vi "12_final.vi"() -> ()   [LabVIEW 2023]
uses:
  <vilib>/Utility/file.llb/Write Delimited Spreadsheet (string).vi
  <vilib>/Utility/file.llb/Read Delimited Spreadsheet (string).vi
panel:
  out "array w/ subset deleted":string[][](array[string])
  out "all rows":string[][](array[string])
  in  "Listbox":i32(listbox)
  in  "stop":bool
  in  "citire":bool
  in  "l":dbl
  in  "L":dbl
  in  "salveaza":bool
  out "XY Graph":cluster{dbl[], dbl[]}(graph)
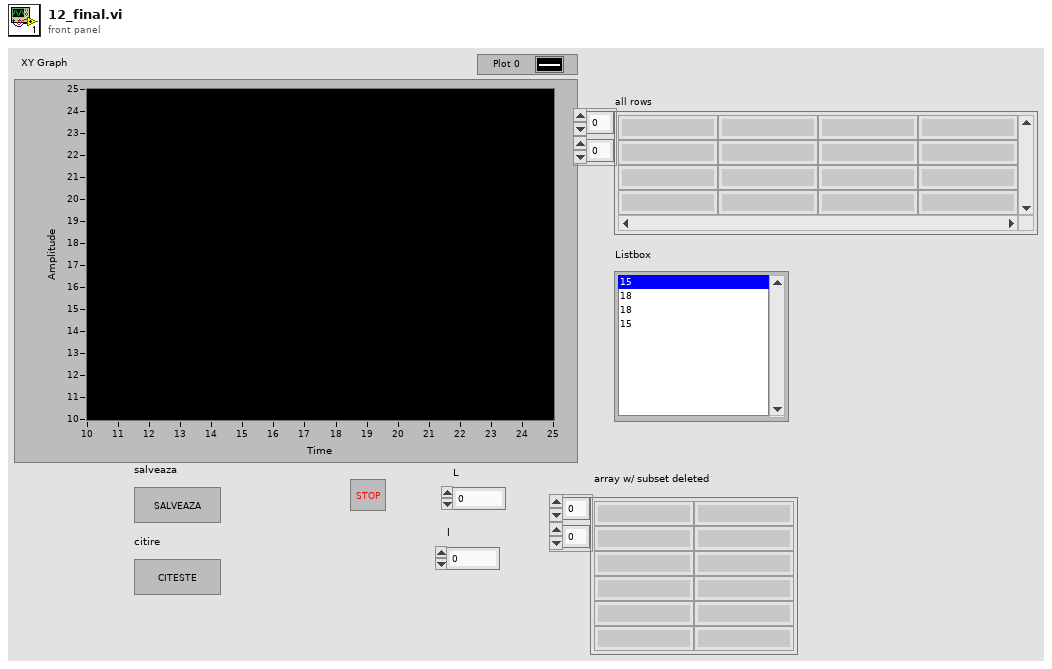
[diagram p1: front panel]
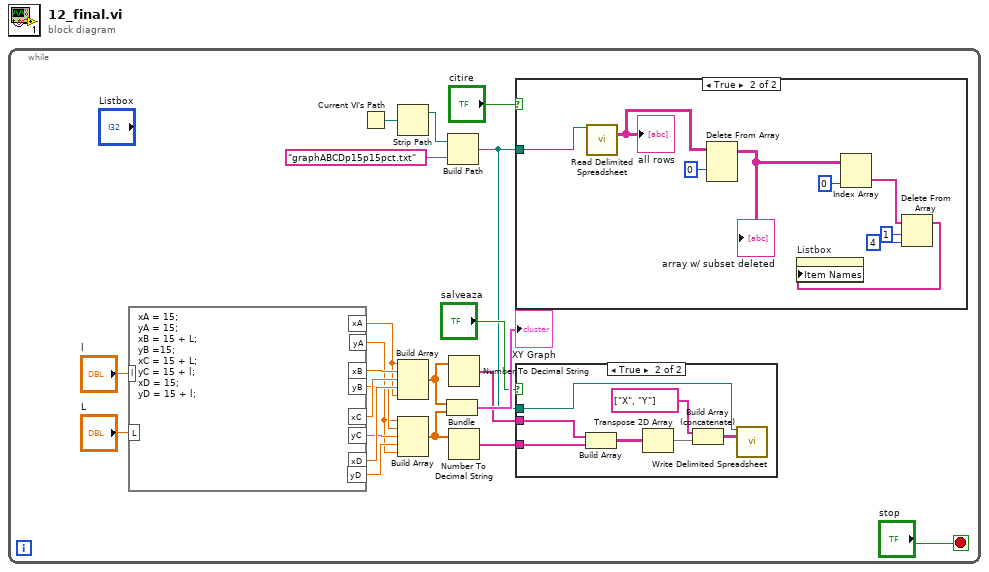
[diagram p0: block diagram]
diagram:
  n1 = while {
    stop <- "stop" stop-if-true
    n2 = formula code="xA = 15;\nyA = 15;\nxB = 15 + L;\nyB =15;\nxC = 15 + L;\nyC = 15 + l;\nxD = 15;\nyD = 15 + l;"("l"="l", "L"="L") -> ("xB"=w20:dbl, "yB"=w17:dbl, "yA"=w13:dbl, "xA"=w14:dbl, "xC"=w19:dbl, "yC"=w16:dbl, "xD"=w18:dbl, "yD"=w15:dbl)
    n3 = Current VI's Path() -> (path=w10:path)
    n4 = Strip Path(path=w10) -> (stripped path=w9:path)  [unwired: 1 out]
    n5 = Build Array(w14, w20, w19, w18, w14) -> (w6:dbl[])
    n6 = Build Array(w13, w17, w16, w15, w13) -> (w4:dbl[])
    n7 = Bundle(w6, w4) -> (→"XY Graph":cluster{dbl[], dbl[]})  [unwired: 1 in]
    n8 = Build Path(base path=w9, name or relative path="graphABCDp15p15pct.txt") -> (appended path=w1:path)
    n9 = Number To Decimal String(number=w6) -> (decimal integer string=w5:string[])  [unwired: 1 in]
    n10 = Number To Decimal String(number=w4) -> (decimal integer string=w3:string[])  [unwired: 1 in]
    n11 = case shown="True" "citire" {
      tunnel: w1 -> [_ w31]
      frame False {
      }
      frame True {
        n12 = call-poly <vilib>:"Read Delimited Spreadsheet.vi"("file path (dialog if empty)"=w31) -> ("all rows"=w30:string[][])  [unwired: 9 in, 5 out]
        "all rows" <- w30
        n13 = Delete From Array(array=w30, index (row)=0) -> (array with subset deleted=w28:string[][])  [unwired: 2 in, 1 out]
        "array w/ subset deleted" <- w28
        n14 = Index Array(array=w28, index (col)=0 ("disabled index (col)")) -> (element=w26:string[])  [unwired: 1 in]
        n15 = Delete From Array(array=w26, length=1, index=4) -> (array with subset deleted=w23:string[])  [unwired: 1 out]
        n16 = property on="Listbox" class="LstBox (strict)"("Item Names"=w23) -> ()  [unwired: 2 in, 2 out]
      }
    }
    n17 = case shown="True" "salveaza" {
      tunnel: w1 -> [_ w38]
      tunnel: w5 -> [_ w37]
      tunnel: w3 -> [_ w36]
      frame False {
      }
      frame True {
        n18 = Build Array(w37, w36) -> (w34:string[][])
        n19 = Transpose 2D Array(2D array=w34) -> (transposed array=w33:string[][])
        n20 = Build Array (concatenate)(string[] ["X", "Y"] ("element"), w33) -> (w32:string[][])
        n21 = call-poly <vilib>:"Write Delimited Spreadsheet.vi"("file path (dialog if empty)"=w38, "2D data"=w32) -> ()  [unwired: 12 in, 2 out]
      }
    }
  }
